vi "TGPPos.vi"(8 "Offset":dbl=182.0, 10 "Angle (-179 - 180)":dbl) -> (2 "TGP Pos":u8)   [LabVIEW 2018]
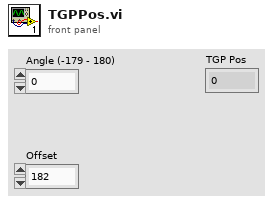
[diagram p1: front panel]
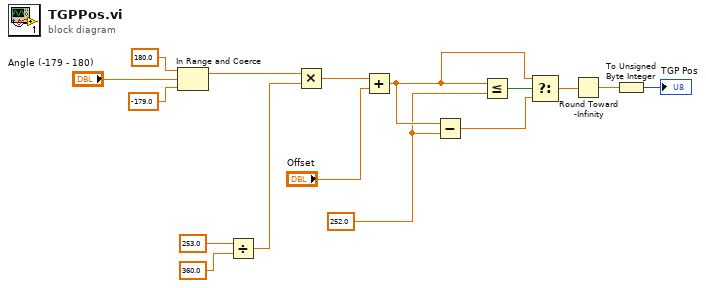
[diagram p0: block diagram]
diagram:
  w4 = 252.0 ("x")
  n1 = In Range and Coerce(upper limit=180.0, x="Angle (-179 - 180)", lower limit=-179.0 ("upper limit")) -> (coerced(x)=w11:dbl)  [unwired: 1 out]
  n2 = Divide(x=253.0, y=360.0 ("x")) -> (x/y=w16:dbl)
  n3 = Multiply(x=w11, y=w16) -> (x*y=w14:dbl)
  n4 = Add(x=w14, y="Offset") -> (x+y=w5:dbl)
  n5 = Subtract(x=w5, y=w4) -> (x-y=w6:dbl)
  n6 = Less Or Equal?(x=w5, y=w4) -> (x <= y?=w7:bool)
  n7 = Select(t=w5, s=w7, f=w6) -> (s? t:f=w3:dbl)
  n8 = Round Toward -Infinity(1:w3) -> (0:w2:dbl)
  n9 = To Unsigned Byte Integer(number=w2) -> (unsigned 8bit integer=→"TGP Pos":u8)
